vi "6221-SR830 scan current(SubVI).vi"(0 "源":i32, 1 "Instrument Ref":refnum<k24>, 2 "Current":dbl=300.0, 3 "Current 2":dbl=300.0, 4 "steps number":i32, 5 "电阻":dbl, 6 "参考信号":T1, 7 "sr830仪器设置":T2={"ID Query (True)"=FALSE, "Reset (True)"=FALSE, "VISA resource name"="", "VISA resource name 2"="", "VISA resource name 3"="", "VISA resource name 4"="", "Sensitivity (-1: Auto gain) 2"=-1, "Sensitivity (-1: Auto gain)"=-1, "量程"=enum."量程每次测量会判定", "SR830 VISA 1"=FALSE, "SR830 VISA 2"=FALSE, "SR830 VISA 3"=FALSE, "SR830 VISA 4"=FALSE, "Sensitivity (-1: Auto gain) 3"=-1, "Sensitivity (-1: Auto gain) 4"=-1, "6221"=FALSE, "6221 resource"="", "2400"=FALSE, "2400 resource"=""} {"Sensitivity (-1: Auto gain) 4" items=["Auto Gain"=-1, "2 nV/fA"=0, "5 nV/fA"=1, "10 nV/fA"=2, "20 nV/fA"=3, "50 nV/fA"=4, "100 nV/fA"=5, "200 nV/fA"=6, "500 nV/fA"=7, "1 uV/pA"=8, "2 uV/pA"=9, "5 uV/pA"=10, "10 uV/pA"=11, "20 uV/pA"=12, "50 uV/pA"=13, "100 uV/pA"=14, "200 uV/pA"=15, "500 uV/pA"=16, "1 mV/nA"=17, "2 mV/nA"=18, "5 mV/nA"=19, "10 mV/nA"=20, "20 mV/nA"=21, "50 mV/nA"=22, "100 mV/nA"=23, "200 mV/nA"=24, "500 mV/mA"=25, "1 V/uA"=26]; "Sensitivity (-1: Auto gain) 3" items=["Auto Gain"=-1, "2 nV/fA"=0, "5 nV/fA"=1, "10 nV/fA"=2, "20 nV/fA"=3, "50 nV/fA"=4, "100 nV/fA"=5, "200 nV/fA"=6, "500 nV/fA"=7, "1 uV/pA"=8, "2 uV/pA"=9, "5 uV/pA"=10, "10 uV/pA"=11, "20 uV/pA"=12, "50 uV/pA"=13, "100 uV/pA"=14, "200 uV/pA"=15, "500 uV/pA"=16, "1 mV/nA"=17, "2 mV/nA"=18, "5 mV/nA"=19, "10 mV/nA"=20, "20 mV/nA"=21, "50 mV/nA"=22, "100 mV/nA"=23, "200 mV/nA"=24, "500 mV/mA"=25, "1 V/uA"=26]; "Sensitivity (-1: Auto gain)" items=["Auto Gain"=-1, "2 nV/fA"=0, "5 nV/fA"=1, "10 nV/fA"=2, "20 nV/fA"=3, "50 nV/fA"=4, "100 nV/fA"=5, "200 nV/fA"=6, "500 nV/fA"=7, "1 uV/pA"=8, "2 uV/pA"=9, "5 uV/pA"=10, "10 uV/pA"=11, "20 uV/pA"=12, "50 uV/pA"=13, "100 uV/pA"=14, "200 uV/pA"=15, "500 uV/pA"=16, "1 mV/nA"=17, "2 mV/nA"=18, "5 mV/nA"=19, "10 mV/nA"=20, "20 mV/nA"=21, "50 mV/nA"=22, "100 mV/nA"=23, "200 mV/nA"=24, "500 mV/mA"=25, "1 V/uA"=26]; "Sensitivity (-1: Auto gain) 2" items=["Auto Gain"=-1, "2 nV/fA"=0, "5 nV/fA"=1, "10 nV/fA"=2, "20 nV/fA"=3, "50 nV/fA"=4, "100 nV/fA"=5, "200 nV/fA"=6, "500 nV/fA"=7, "1 uV/pA"=8, "2 uV/pA"=9, "5 uV/pA"=10, "10 uV/pA"=11, "20 uV/pA"=12, "50 uV/pA"=13, "100 uV/pA"=14, "200 uV/pA"=15, "500 uV/pA"=16, "1 mV/nA"=17, "2 mV/nA"=18, "5 mV/nA"=19, "10 mV/nA"=20, "20 mV/nA"=21, "50 mV/nA"=22, "100 mV/nA"=23, "200 mV/nA"=24, "500 mV/mA"=25, "1 V/uA"=26]}, 15 "队列输入":refnum<queue>, 19 "abort":refnum<queue>) -> (17 "错误输出":errorcluster, 18 "电压":dbl)   [LabVIEW 2019, in "SubVI.lvlib"]
uses:
  SubVI.lvlib
  measure/lib/QDInstrument.dll
  Keithley 622x/Keithley 622x.lvlib
panel:
  out "数组":dbl[](array[numeric])
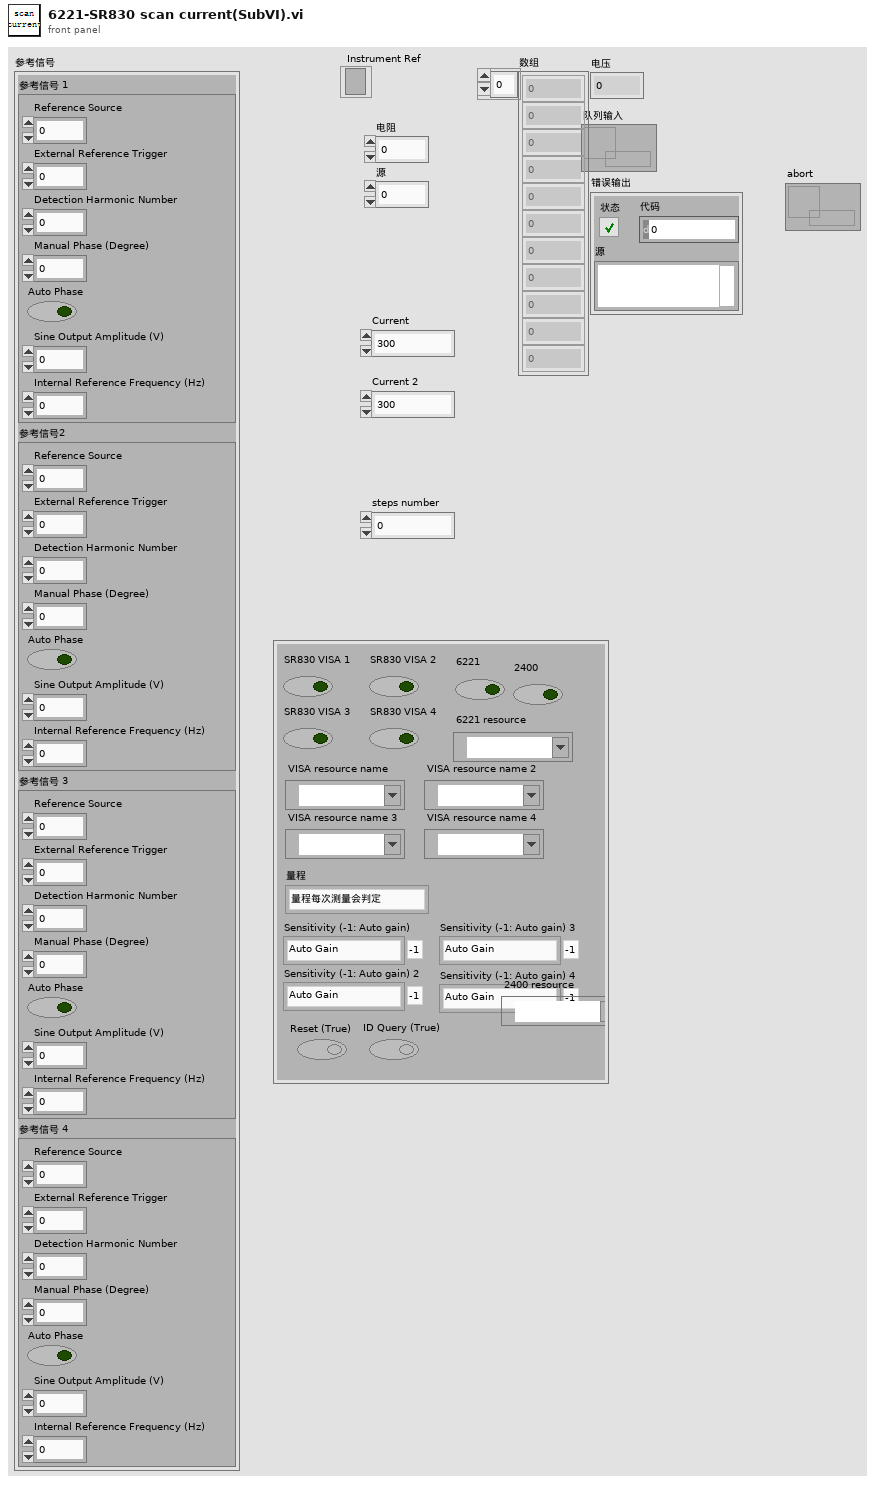
[diagram p1: front panel]
types:
  T1 = cluster{"参考信号 1":cluster{"Reference Source":u16, "External Reference Trigger  ":u16, "Detection Harmonic Number ":dbl, "Manual Phase (Degree)":dbl, "Auto Phase ":bool, "Sine Output Amplitude (V)":dbl, "Internal Reference Frequency (Hz)":dbl}, "参考信号2":cluster{"Reference Source":u16, "External Reference Trigger  ":u16, "Detection Harmonic Number ":dbl, "Manual Phase (Degree)":dbl, "Auto Phase ":bool, "Sine Output Amplitude (V)":dbl, "Internal Reference Frequency (Hz)":dbl}, "参考信号 3":cluster{"Reference Source":u16, "External Reference Trigger  ":u16, "Detection Harmonic Number ":dbl, "Manual Phase (Degree)":dbl, "Auto Phase ":bool, "Sine Output Amplitude (V)":dbl, "Internal Reference Frequency (Hz)":dbl}, "参考信号 4":cluster{"Reference Source":u16, "External Reference Trigger  ":u16, "Detection Harmonic Number ":dbl, "Manual Phase (Degree)":dbl, "Auto Phase ":bool, "Sine Output Amplitude (V)":dbl, "Internal Reference Frequency (Hz)":dbl}}
  T2 = cluster{"ID Query (True)":bool, "Reset (True)":bool, "VISA resource name":refnum<visa-resource-name>, "VISA resource name 2":refnum<visa-resource-name>, "VISA resource name 3":refnum<visa-resource-name>, "VISA resource name 4":refnum<visa-resource-name>, "Sensitivity (-1: Auto gain) 2":i16, "Sensitivity (-1: Auto gain)":i16, "量程":enum16{"量程每次测量会判定", "量程不变为设定值"}, "SR830 VISA 1":bool, "SR830 VISA 2":bool, "SR830 VISA 3":bool, "SR830 VISA 4":bool, "Sensitivity (-1: Auto gain) 3":i16, "Sensitivity (-1: Auto gain) 4":i16, "6221":bool, "6221 resource":refnum<visa-resource-name>, "2400":bool, "2400 resource":refnum<visa-resource-name>}
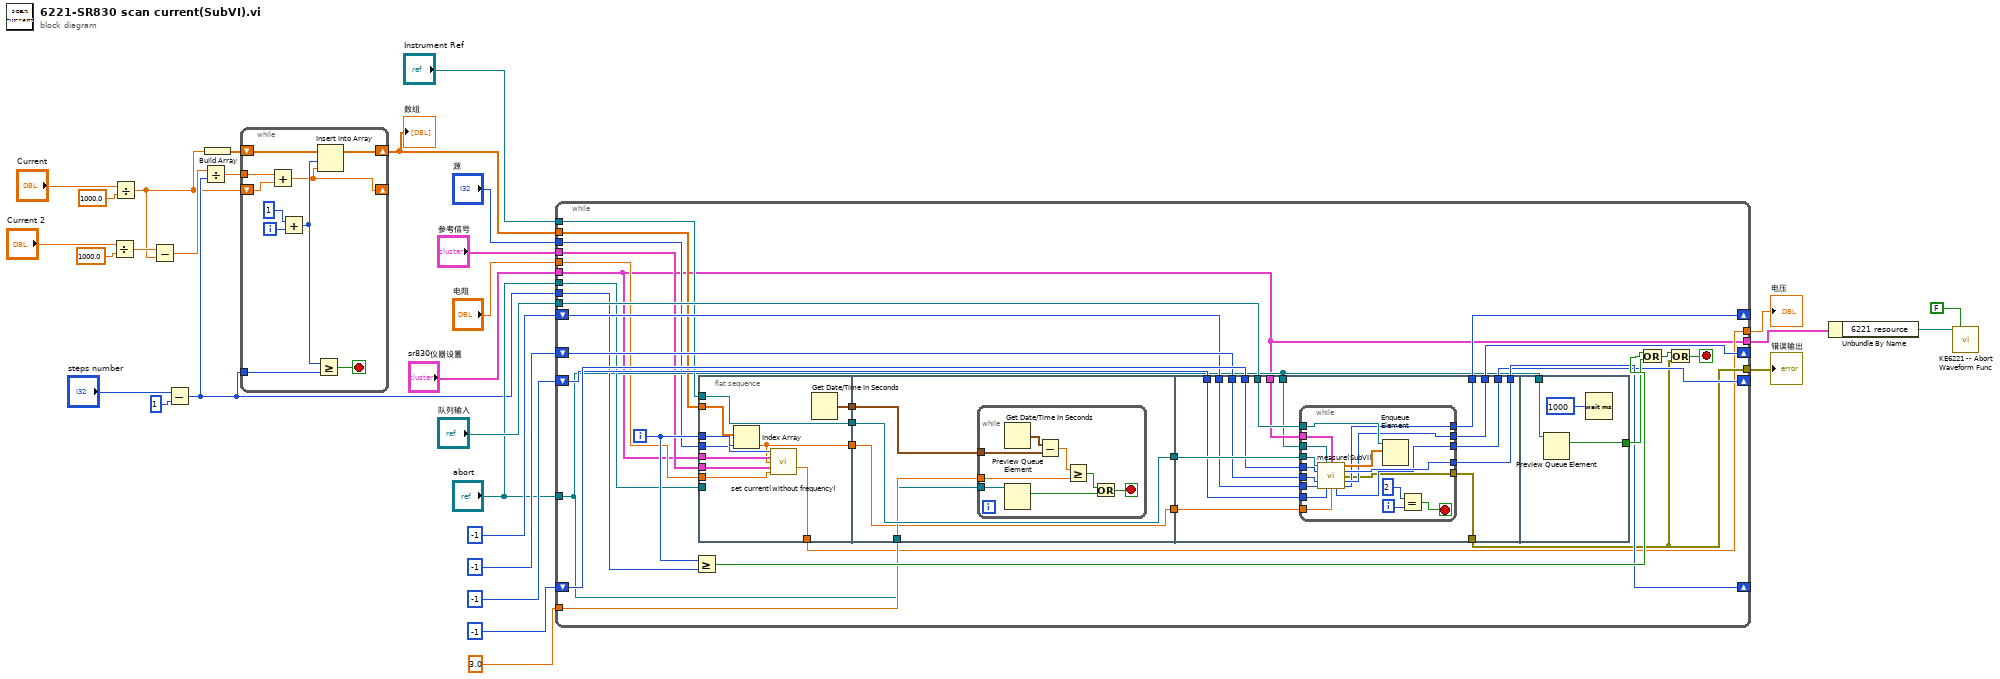
[diagram p0: block diagram]
diagram:
  n1 = Divide(x="Current 2", y=1000.0) -> (x/y=w9:dbl)
  n2 = Divide(x="Current", y=1000.0) -> (x/y=w5:dbl)
  n3 = Subtract(x=w9, y=w5) -> (x-y=w28:dbl)
  n4 = Subtract(x="steps number", y=1) -> (x-y=w15:i32)
  n5 = Divide(x=w28, y=w15) -> (x/y=w30:dbl)
  n6 = Build Array(w5) -> (w29:dbl[])
  n7 = while {
    shift-right: [w40] -> w23
    shift-left: w29 -> [w39]
    tunnel: w30 -> [w34]
    tunnel: w15 -> [w33]
    shift-right: [w32] -> _
    shift-left: w5 -> [w31]
    i -> [w38]
    stop <- w35 stop-if-true
    n8 = Add(x=w34, y=w31) -> (x+y=w32:dbl)
    n9 = Add(x=1, y=w38) -> (x+y=w36:i32)
    n10 = Greater Or Equal?(x=w36, y=w33) -> (x >= y?=w35:bool)
    n11 = Insert Into Array(array=w39, index=w36, new element=w32) -> (w40:dbl[])
  }
  "数组" <- w23
  n12 = while {
    tunnel: w15 -> [w60]
    tunnel: "队列输入" -> [w71]
    tunnel: "abort" -> [w49]
    shift-right: [w67] -> _
    shift-left: -1 ("量程结束") -> [w68]
    shift-right: [w65] -> _
    shift-left: -1 ("量程结束") -> [w66]
    shift-right: [w63] -> _
    shift-left: -1 ("量程结束") -> [w64]
    shift-right: [w62] -> _
    shift-left: -1 ("量程结束") -> [w61]
    tunnel: "Instrument Ref" -> [w58]
    tunnel: w23 -> [w57]
    tunnel: "sr830仪器设置" -> [w41]
    tunnel: "abort" -> [w56]
    tunnel: [w53] -> w18
    tunnel: 3.0 ("Delay") -> [w50]
    tunnel: "电阻" -> [w47]
    tunnel: "源" -> [w46]
    tunnel: "参考信号" -> [w45]
    tunnel: [w42] -> w11
    tunnel: [w41] -> w3
    i -> [w59]
    stop <- w54 stop-if-true
    n13 = Greater Or Equal?(x=w59, y=w60) -> (x >= y?=w70:bool)
    n14 = flat-sequence {
      tunnel: w59 -> [w80]
      tunnel: w58 -> [w78]
      tunnel: w57 -> [w81]
      tunnel: w56 -> [_]
      tunnel: [w79] -> w51
      tunnel: [w78] -> w48
      tunnel: w41 -> [w77]
      tunnel: w47 -> [w73]
      tunnel: w46 -> [w76]
      tunnel: w45 -> [w75]
      tunnel: [w74] -> w44
      tunnel: [w72] -> w42
      tunnel: [w86] -> w52
      tunnel: w51 -> [w85]
      tunnel: w50 -> [w84]
      tunnel: w49 -> [w83]
      tunnel: w48 -> [w86]
      tunnel: w44 -> [w82]
      tunnel: [w82] -> w43
      tunnel: w52 -> [w108]
      tunnel: w71 -> [w107]
      tunnel: w68 -> [w98]
      tunnel: [w106] -> w67
      tunnel: w66 -> [w105]
      tunnel: [w104] -> w65
      tunnel: w64 -> [w103]
      tunnel: [w102] -> w63
      tunnel: [w101] -> w62
      tunnel: w61 -> [w100]
      tunnel: w41 -> [w99]
      tunnel: w49 -> [w97]
      tunnel: [w96] -> w53
      tunnel: w43 -> [w95]
      tunnel: w49 -> [w129]
      tunnel: [w128] -> w69
      frame #0 {
        n15 = Index Array(array=w81, index=w80) -> (element=w74:dbl)
        n16 = call "set current(without frequency).vi"("源"=w76, "仪器设置"=w77, "电流"=w74, "参考信号"=w75, "电阻"=w73) -> ("电流/电压"=w72:dbl)  [unwired: 10 in]
        n17 = Get Date/Time In Seconds() -> (seconds since 1Jan1904=w79:timestamp)
      }
      frame #1 {
        n18 = while {
          tunnel: w85 -> [w93]
          tunnel: w84 -> [w91]
          tunnel: w83 -> [w89]
          stop <- w87 stop-if-true
          n19 = Get Date/Time In Seconds() -> (seconds since 1Jan1904=w94:timestamp)
          n20 = Preview Queue Element(queue=w89) -> (element=w88:bool)  [unwired: 2 in, 3 out]
          n21 = Subtract(x=w94, y=w93) -> (x-y=w92:dbl)
          n22 = Greater Or Equal?(x=w92, y=w91) -> (x >= y?=w90:bool)
          n23 = Or(x=w90, y=w88) -> (x .or. y?=w87:bool)
        }
      }
      frame #2 {
        n24 = while {
          tunnel: w108 -> [w126]
          tunnel: w107 -> [w125]
          tunnel: [w123] -> w106
          tunnel: w105 -> [w122]
          tunnel: [w121] -> w104
          tunnel: w103 -> [w120]
          tunnel: [w119] -> w102
          tunnel: [w118] -> w101
          tunnel: w100 -> [w117]
          tunnel: w99 -> [w116]
          tunnel: w98 -> [w115]
          tunnel: w97 -> [w114]
          tunnel: [w113] -> w96
          tunnel: w95 -> [w109]
          i -> [w112]
          stop <- w110 stop-if-true
          n25 = call "measure(SubVI).vi"(".NET引用句柄输入"=w126, "abort"=w114, "sr830仪器设置"=w116, "量程入 1"=w115, "量程入 2"=w122, "量程入 3"=w120, "量程入 4"=w117, "电流"=w109) -> ("数组"=w124:dbl[], "量程出 1"=w123:i32, "错误输出"=w113:errorcluster, "量程出 2"=w121:i32, "量程出 4"=w118:i32, "量程出 3"=w119:i32)  [unwired: 2 in]
          n26 = Enqueue Element(queue=w125, element=w124) -> ()  [unwired: 2 in, 3 out]
          n27 = Equal?(x=2, y=w112) -> (x = y?=w110:bool)
        }
      }
      frame #3 {
        n28 = Preview Queue Element(queue=w129) -> (element=w128:bool)  [unwired: 2 in, 3 out]
        n29 = Wait (ms)(milliseconds to wait=u32 1000 ("等待时间（毫秒）")) -> ()  [unwired: 1 out]
      }
    }
    n30 = Or(x=w70, y=w69) -> (x .or. y?=w55:bool)
    n31 = Or(x=w55, y=w53) -> (x .or. y?=w54:bool)
  }
  "错误输出" <- w18
  "电压" <- w11
  n32 = Unbundle By Name(w3) -> ("6221 resource"=w2:refnum<visa-resource-name>)
  n33 = call "KE6221 -- Abort Waveform Func.vi"("Resource In"=w2, "Check For SCPI Errors? (T)"=FALSE) -> ()  [unwired: 12 in, 2 out]
